vi "convert binary to signal.vi"(8 "Binary CJC":u32, 9 "Thermocouple data?":bool, 10 "Binary raw":i32, 11 "Voltage Range":T1 items=["+/- 60V", "+/- 15V", "+/- 4V", "+/- 1V", "+/- 125mV"]) -> (0 "R_T":sgl, 3 "signal":sgl)   [LabVIEW 2018]
uses:
  Type Def Ctrls/FPGA ctrls/NI9219VoltageRange.ctl
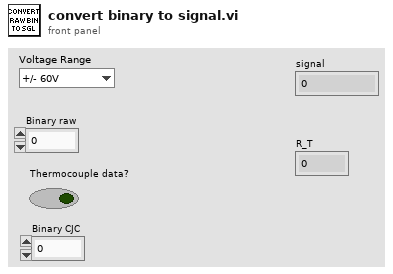
[diagram p1: front panel]
types:
  T1 = typedef "NI9219VoltageRange.ctl" = u8
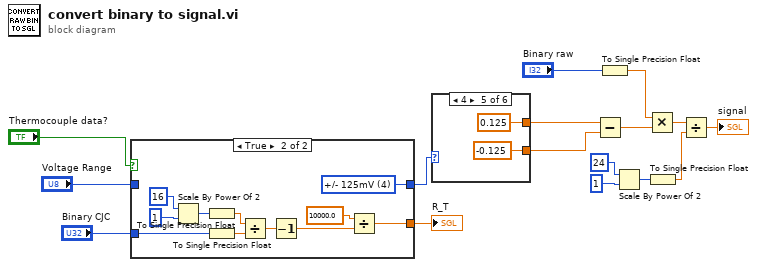
[diagram p0: block diagram]
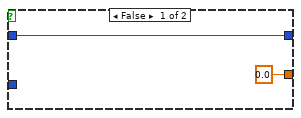
[diagram p2: hidden frame]
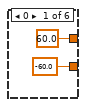
[diagram p3: hidden frame]
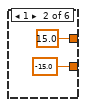
[diagram p4: hidden frame]
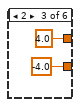
[diagram p5: hidden frame]
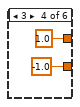
[diagram p6: hidden frame]
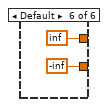
[diagram p7: hidden frame]
diagram:
  n1 = case shown="True" "Thermocouple data?" {
    tunnel: [sgl 0.0 w26] -> w9
    tunnel: "Voltage Range" -> [w17 _]
    tunnel: [w17 w23] -> w7
    tunnel: "Binary CJC" -> [_ w22]
    frame False {
    }
    frame True {
      w23 = T1 4 items=["+/- 60V", "+/- 15V", "+/- 4V", "+/- 1V", "+/- 125mV"] ("Voltage Range")
      n2 = Scale By Power Of 2(n=i16 16 ("y"), x=u32 1) -> (x*2^n=w19:u32)
      n3 = To Single Precision Float(number=w19) -> (single precision float=w25:sgl)
      n4 = To Single Precision Float(number=w22) -> (single precision float=w24:sgl)
      n5 = Divide(x=w25, y=w24) -> (x/y=w29:sgl)
      n6 = Decrement(x=w29) -> (x-1=w27:sgl)
      n7 = Divide(x=sgl 10000.0, y=w27) -> (x/y=w26:sgl)
    }
  }
  "R_T" <- w9
  n8 = case shown="4" w7 {
    tunnel: [sgl 60.0 sgl 15.0 sgl 4.0 sgl 1.0 sgl 0.125 sgl inf] -> w16
    tunnel: [sgl -60.0 sgl -15.0 sgl -4.0 sgl -1.0 sgl -0.125 sgl -inf] -> w15
    frame 0 {
    }
    frame 1 {
    }
    frame 2 {
    }
    frame 3 {
    }
    frame 4 {
    }
    frame Default {
    }
  }
  n9 = Subtract(x=w16, y=w15) -> (x-y=w14:sgl)
  n10 = To Single Precision Float(number="Binary raw") -> (single precision float=w6:sgl)
  n11 = Scale By Power Of 2(n=i16 24 ("y"), x=u32 1) -> (x*2^n=w2:u32)
  n12 = Multiply(x=w6, y=w14) -> (x*y=w12:sgl)
  n13 = To Single Precision Float(number=w2) -> (single precision float=w1:sgl)
  n14 = Divide(x=w12, y=w1) -> (x/y=→"signal":sgl)
